vi "Call VI API.vi"(8 "error in":errorcluster, 10 "Section":string, 11 "DVR In":refnum<data-value>) -> (0 "error out":errorcluster, 1 "VI Ref":refnum<vi>, 2 "Asynch Ref":refnum<vi>, 3 "DVR Out":refnum<data-value>)   [LabVIEW 2020, in "Speed Mode.lvclass"]
uses:
  Speed Mode.lvclass
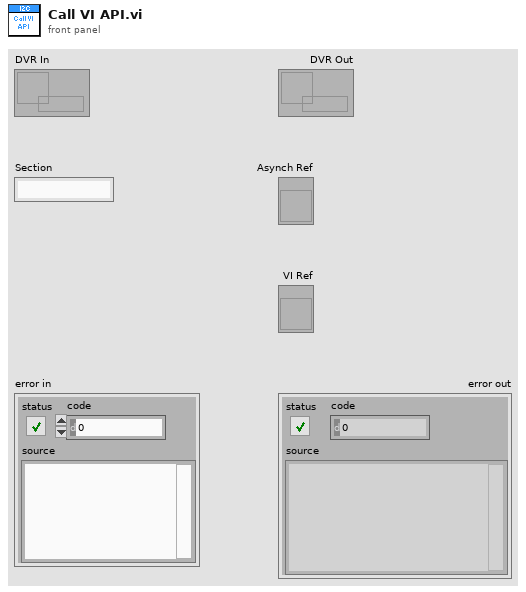
[diagram p1: front panel]
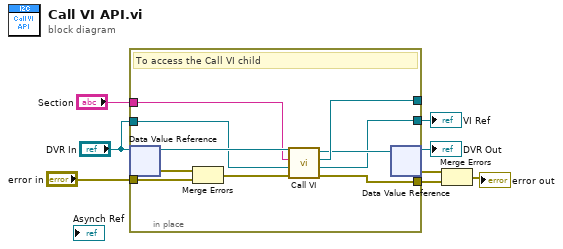
[diagram p0: block diagram]
diagram:
  n1 = in-place {
    in-place-border: "Section" -> [w17]
    in-place-border: "error in" -> [w14]
    in-place-border: [w13] -> _
    in-place-border: [w12] -> w5
    in-place-border: [w10] -> w2
    in-place-border: "DVR In" -> [w9]
    # "To access the Call VI child"
    n2 = in-place-dvr #1("DVR In") -> (w18:refnum<class "Speed Mode.lvclass">, w16:errorcluster)
    n3 = Merge Errors(w16, w14) -> (w15:errorcluster)
    n4 = call-dynamic "Call VI.vi"("error in (no error)"=w15, "DVR"=w9, "Section"=w17, "Speed Mode in"=w18) -> ("error out"=w12:errorcluster, "VI Ref"=w10:refnum<vi>, "Asynch Ref"=w13:refnum<vi>, "Speed Mode out"=w11:refnum<class "Speed Mode.lvclass">)  [unwired: 4 in]
    n5 = in-place-dvr #1(w11) -> (→"DVR Out":refnum<data-value>, w6:errorcluster)
  }
  "VI Ref" <- w2
  n6 = Merge Errors(w6, w5) -> (→"error out":errorcluster)
